vi "split_error.vi"(8 "error in":errorcluster) -> (0 "error out":errorcluster, 1 "callStack":string, 2 "Location":string, 3 "Details":string)   [LabVIEW 2023]
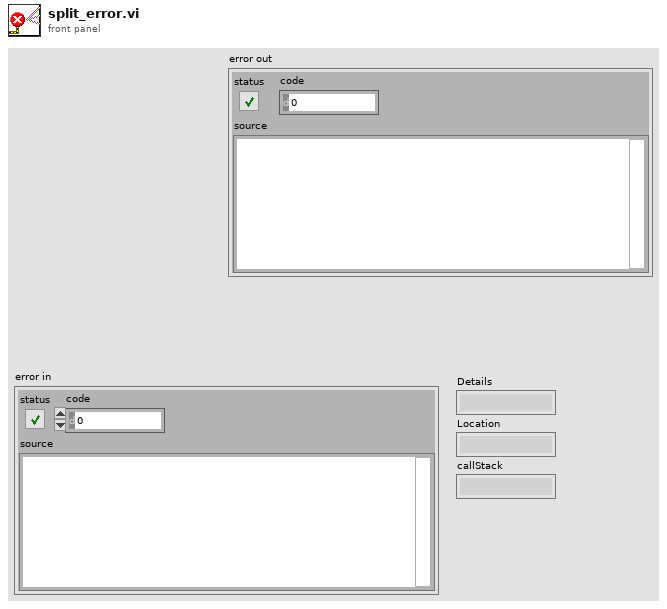
[diagram p1: front panel]
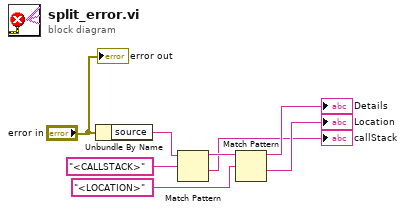
[diagram p0: block diagram]
diagram:
  n1 = Unbundle By Name("error in") -> ("source"=w8:string)
  n2 = Match Pattern(string=w8, regular expression="<CALLSTACK>" ("string")) -> (before substring=w4:string, after substring=→"callStack":string)  [unwired: 1 in, 2 out]
  n3 = Match Pattern(string=w4, regular expression="<LOCATION>" ("string")) -> (before substring=→"Details":string, after substring=→"Location":string)  [unwired: 1 in, 2 out]
  "error out" <- "error in"
